vi "CRYAuto Save.vi"(0 "Setup in":T1={"No.VI"=0, "Category"="", "StepName"="", "Seq setup flattened"="", "Comment"="", "Steps config."=[], "Jump config"=[], "Start"=0.0, "Increment"=0.0, "Name"="Pa", "Unit"="Pa", "Y data"=1, "Y prefix"="", "Y dB ref"=1.0, "Y unit"="", "Repeat State Array"=[]} {"Repeat State Array"."Start" format="%#_5g"; "Y dB ref" format="%.1f"; "Y data" items=["dB", "Lin"]; "Start" format="%#_5g"}, 5 "Data in":T6 {"Z data" items=["dB", "Lin"]; "X data" items=["dB", "Lin"]; "Y data" items=["dB", "Lin"]; "Z dB ref" format="%.1f"; "Z axis" items=["Log", "Lin"]; "X dB ref" format="%.1f"; "X axis" items=["Log", "Lin"]; "Y axis" items=["Log", "Lin"]; "Y dB ref" format="%.1f"; "Curve"."z" format="%.2f"; "Curve"."y" format="%.2f"; "Curve"."x" format="%.2f"}, 7 "Results in":T2 {"Margin" format="%.2f"}, 9 "Seq Setup in":string, 11 "Step name":string, 12 "Hardware in":string, 13 "Calibration in":string) -> (3 "Types Out":string[](array[string]), 4 "Inserted Names Out":string[](array[string]), 6 "Data out":T6 {"Z data" items=["dB", "Lin"]; "X data" items=["dB", "Lin"]; "Y data" items=["dB", "Lin"]; "Z dB ref" format="%.1f"; "Z axis" items=["Log", "Lin"]; "X dB ref" format="%.1f"; "X axis" items=["Log", "Lin"]; "Y axis" items=["Log", "Lin"]; "Y dB ref" format="%.1f"; "Curve"."z" format="%.2f"; "Curve"."y" format="%.2f"; "Curve"."x" format="%.2f"}, 8 "Results out":T2 {"Margin" format="%.2f"}, 10 "Wave out":T4 {"Y dB ref" format="%.1f"; "Y axis" items=["Log", "Lin"]; "Y data" items=["dB", "Lin"]; "X data" items=["dB", "Lin"]})   [LabVIEW 2013]
uses:
  Typedef Control/CRYData Cluster Array.ctl
  Typedef Control/CRYData Cluster.ctl
  Typedef Control/CRYResult Cluster Array.ctl
  Typedef Control/CRYResult Cluster.ctl
  Typedef Control/CRYWaveform Cluster Array.ctl
  Typedef Control/CRYWaveform Cluster.ctl
  Typedef Control/CRYStep.ctl
  Data/CRYData & result stacks global.vi
  CRYMainGlobal.vi
  Calibration/SubVI/CRYCal Global.vi
  CRYProject/CRYProject Editor Global.vi
panel:
  out "Channel":i32
  out "filepath":string caption="Saving to file:"
  in  "Display Step":bool=TRUE
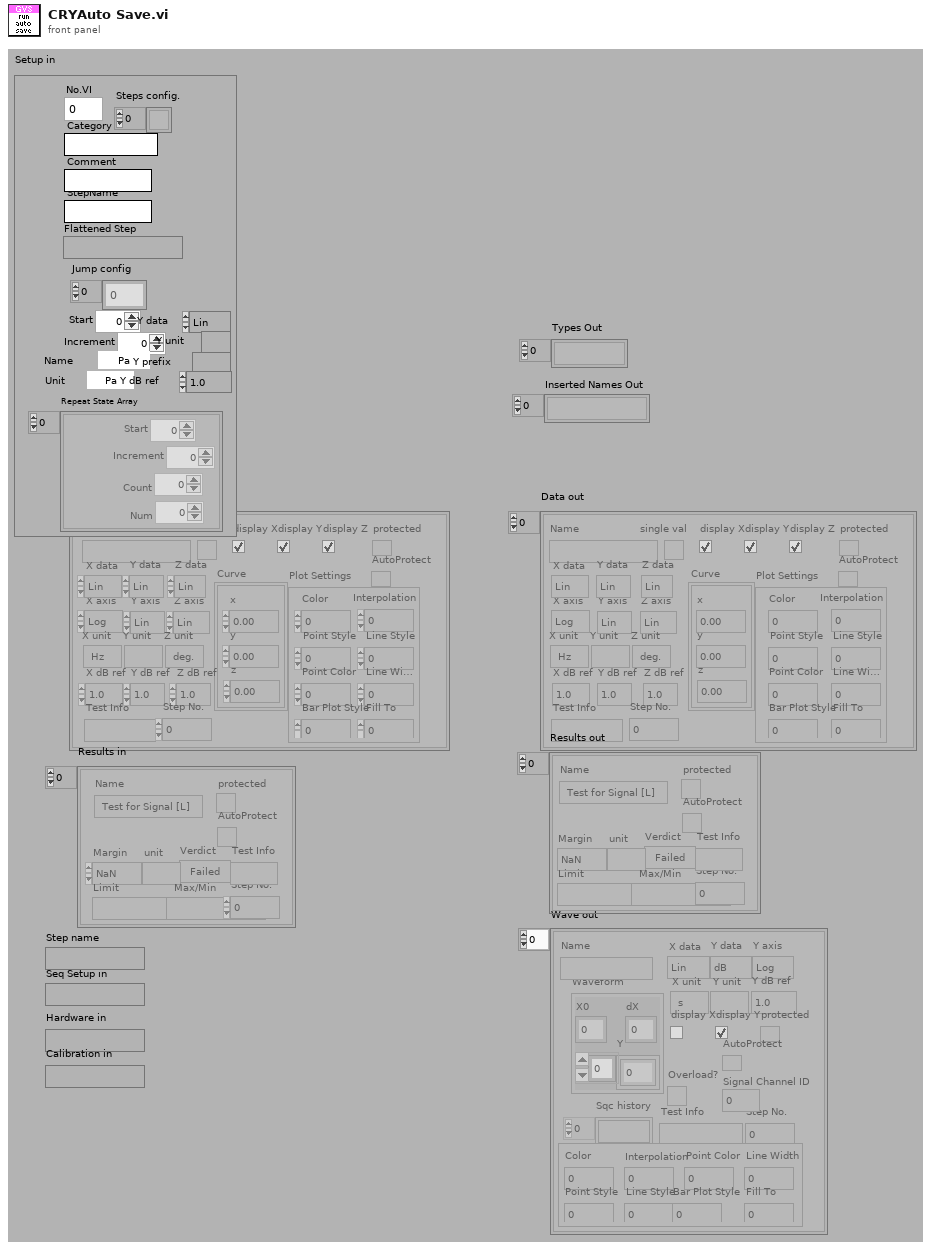
[diagram p1: front panel]
types:
  T1 = typedef "CRYStep.ctl" = cluster{"No.VI":i32, "Category":string, "StepName":string, "Seq setup flattened":string, "Comment":string, "Steps config.":bool[], "Jump config":i32[], "Start":dbl, "Increment":dbl, "Name":string, "Unit":string, "Y data":u16, "Y prefix":string, "Y dB ref":dbl, "Y unit":string, "Repeat State Array":cluster{"Start":dbl, "Increment":dbl, "Count":i32, "Num":i32}[]}
  T2 = typedef "CRYResult Cluster Array.ctl" = T3[]
  T3 = typedef "CRYResult Cluster.ctl" = cluster{"Name":string, "Margin":dbl, "unit":string, "Verdict":bool, "Limit":string, "Max/Min":string, "protected":bool, "Step No.":i32, "Test Info":string, "AutoProtect":bool}
  T4 = typedef "CRYWaveform Cluster Array.ctl" = T5[]
  T5 = typedef "CRYWaveform Cluster.ctl" = cluster{"Waveform":cluster{"X0":dbl, "dX":dbl, "Y":sgl[]}, "X data":u16, "Y data":u16, "Y axis":u16, "X unit":string, "Y unit":string, "Y dB ref":dbl, "display Y":bool, "display X":bool, "Overload?":bool, "Test Info":string, "Step No.":i32, "Name":string, "protected":bool, "Sqc history":string[], "Signal Channel ID":i32, "Plot Settings":cluster{"Color":u32, "Interpolation":u8, "Point Style":u8, "Line Style":u8, "Point Color":u32, "Line Width":u8, "Bar Plot Style":u8, "Fill To":i16}, "AutoProtect":bool}
  T6 = typedef "CRYData Cluster Array.ctl" = T7[]
  T7 = typedef "CRYData Cluster.ctl" = cluster{"Name":string, "Curve":cluster{"x":dbl, "y":dbl, "z":dbl}[], "X data":u16, "Y data":u16, "Z data":u16, "X axis":u16, "Y axis":u16, "Z axis":u16, "X unit":string, "Y unit":string, "Z unit":string, "X dB ref":dbl, "Y dB ref":dbl, "Z dB ref":dbl, "single val":bool, "protected":bool, "display X":bool, "display Y":bool, "display Z":bool, "Test Info":string, "Step No.":i32, "Plot Settings":cluster{"Color":u32, "Interpolation":u8, "Point Style":u8, "Line Style":u8, "Point Color":u32, "Line Width":u8, "Bar Plot Style":u8, "Fill To":i16}, "AutoProtect":bool}
  T8 = enum16{"OK", "Yes", "YesNo", "YesNoCancel", "ReplaceAppend"}
  T9 = typedef "CRYAuto Save Cluster.ctl" = cluster{"Name":string, "save":enum16{"Data", "Results", "Waveforms"}, "Item Names":string[], "Autosave folder":path, "data format":u16, "filename option":enum16{"auto", "prompt"}, "fn construction":i32[], "layout":enum16{"rows", "columns"}, "notation":enum16{"sci", "float"}, "precision":i32, "prompt comment":bool, "header":enum16{"none", "standard", "custom"}, "custom header":string, "serial no.":bool, "User defined":string, "delimiter":enum16{"tab", "comma", "space", "other"}, "other delim":string, "axes":cluster{"x":bool, "y":bool, "z":bool}, "Time Stamp":bool, "Lot No.":bool, "Operator":bool, "Excel Template":string, "New or Append":u16, "Data":u16, "Help":string, "Tab Value":enum32{"Setting", "Help"}, "UDL or DSN":path, "User Default":bool, "Selector":i32, "Axis":u16, "Value Name":string, "format string":cluster{"dB Format String out":string, "Lin Format String out":string}, "DBPath":path}
  T10 = cluster{"dB Format String out":string, "Lin Format String out":string}
  T11 = cluster{"layout":enum16{"rows", "columns"}, "notation":enum16{"sci", "float"}, "precision":i32, "header":enum16{"none", "standard", "custom"}, "custom header":string, "serial no.":bool, "delimiter":enum16{"tab", "comma", "space", "other"}, "other delim":string, "axes":cluster{"x":bool, "y":bool, "z":bool}, "Lot No.":bool, "Operator":bool, "Time Stamp":bool}
  T12 = typedef "CRYTS.ctl" = cluster{"No.TS":u16, "TS File Path":path, "TS Name":string, "EditStepName":string, "Steps":T1[], "New State":bool, "Change State":bool, "Flattened CurveLib Data":string, "Document Data":string, "EditStepNo":u16, "Operator Start File":string, "Sequence Type":string, "Sequence Language":string}
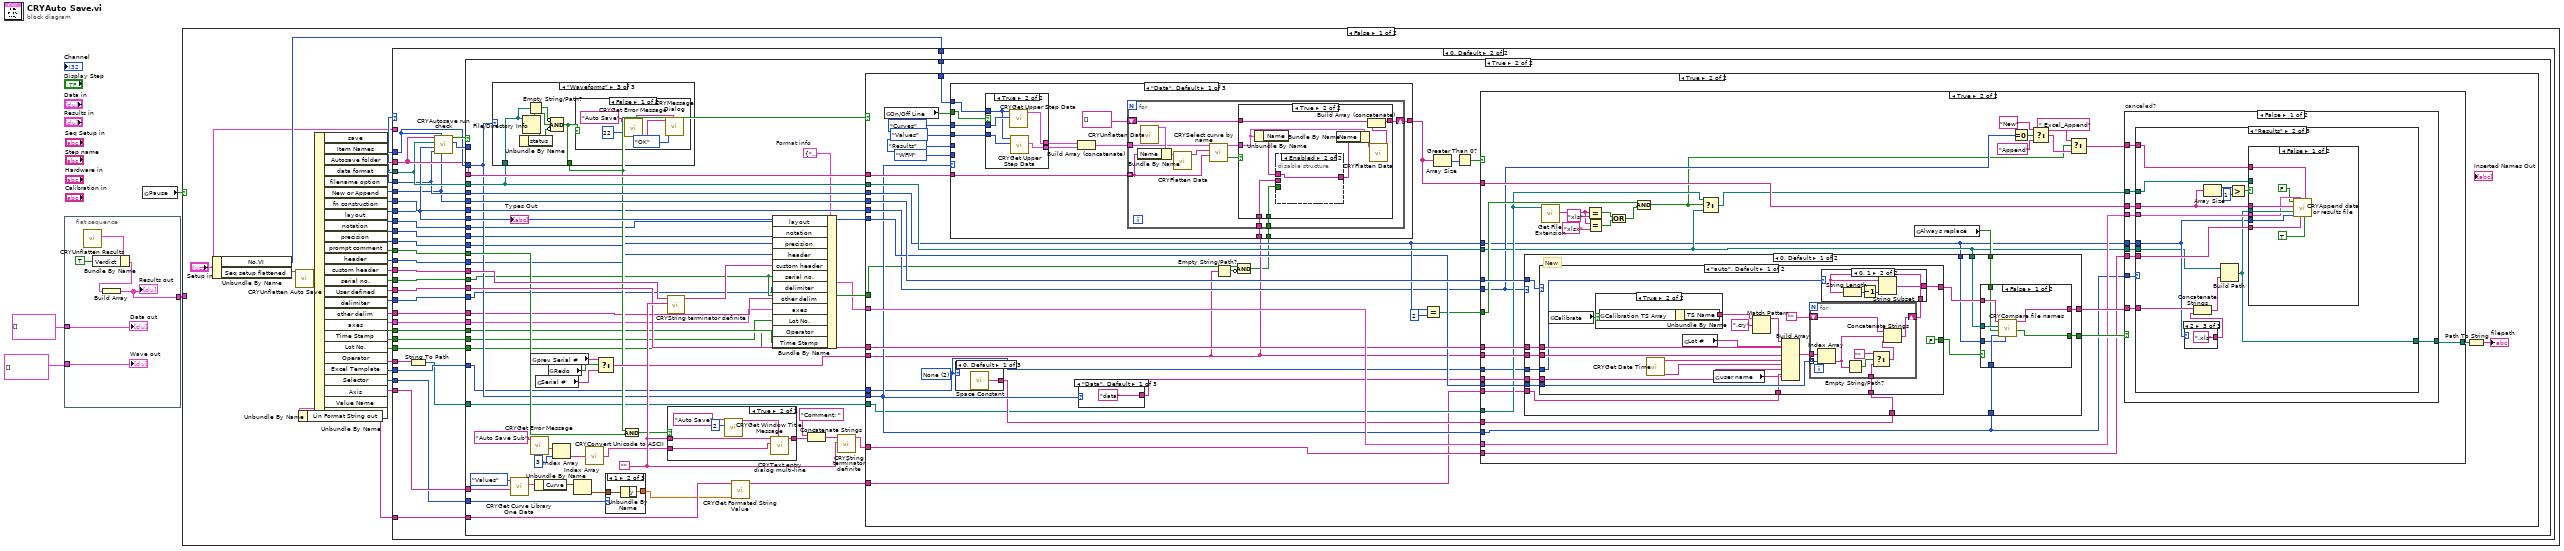
[diagram p0: block diagram]
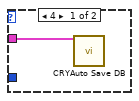
[diagram p2: hidden frame]
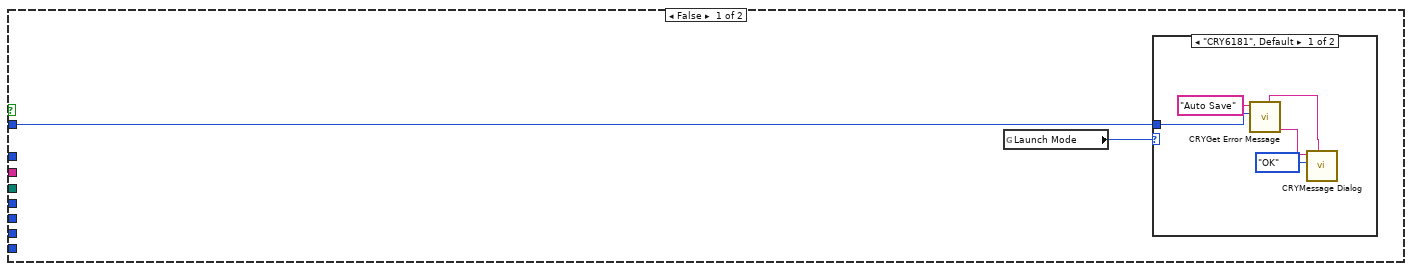
[diagram p3: hidden frame]
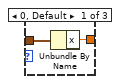
[diagram p5: hidden frame]
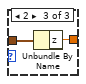
[diagram p6: hidden frame]
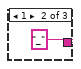
[diagram p8: hidden frame]
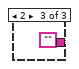
[diagram p9: hidden frame]
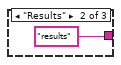
[diagram p10: hidden frame]
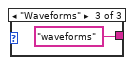
[diagram p11: hidden frame]
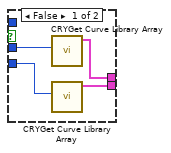
[diagram p12: hidden frame]
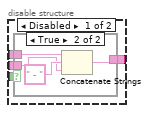
[diagram p14: hidden frame]
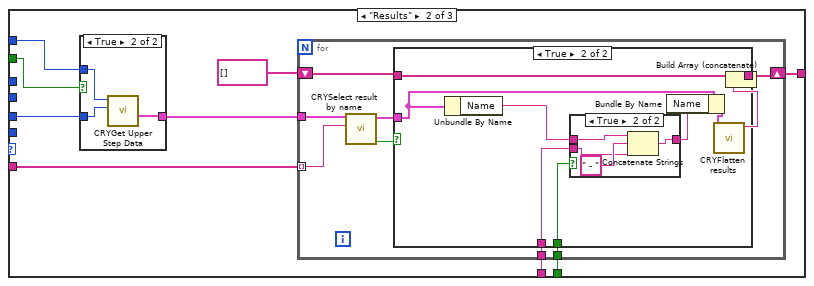
[diagram p16: hidden frame]
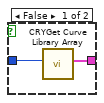
[diagram p17: hidden frame]
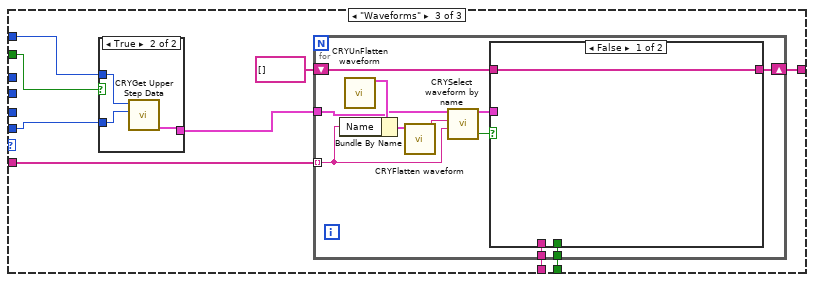
[diagram p20: hidden frame]
diagram:
  n1 = flat-sequence {
    tunnel: T6 [] ("Data out") -> [w7]
    tunnel: [w6] -> w3
    tunnel: T4 [] ("Wave out") -> [w5]
    frame #0 {
      n2 = call "CRYUnflatten Results.vi"() -> ("Result"=w10:T3)  [unwired: 9 in, 2 out]
      n3 = Bundle By Name(cluster=w10, "Verdict"=TRUE) -> (w8:T3)
      n4 = Build Array(w8) -> (w6:T3[])
      "Results out" <- w6
      "Data out" <- w7
      "Wave out" <- w5
    }
  }
  n5 = global read "CRYData & result stacks global.vi" "Pause"() -> (w2:bool)
  n6 = case shown="False" w2 {
    tunnel: w3 -> [_ _]
    frame False {
      n7 = Unbundle By Name("Setup in") -> ("No.VI"=w13:i32, "Seq setup flattened"=w20:string)
      n8 = call "CRYUnflatten Auto Save.vi"("Flatten Auto Save"=w20) -> ("Auto save"=w30:T9)  [unwired: 8 in, 2 out]
      n9 = Unbundle By Name(w30) -> ("save"=w25:enum16{"Data", "Results", "Waveforms"}, "Item Names"=w24:string[], "Autosave folder"=w23:path, "data format"=w12:u16, "filename option"=w21:enum16{"auto", "prompt"}, "New or Append"=w26:u16, "fn construction"=w22:i32[], "layout"=w38:enum16{"rows", "columns"}, "notation"=w39:enum16{"sci", "float"}, "precision"=w40:i32, "prompt comment"=w36:bool, "header"=w41:enum16{"none", "standard", "custom"}, "custom header"=w37:string, "serial no."=w34:bool, "User defined"=w35:string, "delimiter"=w33:enum16{"tab", "comma", "space", "other"}, "other delim"=w32:string, "axes"=w31:cluster{"x":bool, "y":bool, "z":bool}, "Time Stamp"=w29:bool, "Lot No."=w28:bool, "Operator"=w27:bool, "Excel Template"=w18:string, "Selector"=w19:i32, "Axis"=w16:u16, "Value Name"=w17:string, "format string"=w15:T10)
      n10 = Unbundle By Name(w15) -> ("Lin Format String out"=w14:string)
      n11 = case shown="0, Default" w12 {
        tunnel: w41 -> [_ w72]
        tunnel: w40 -> [_ w71]
        tunnel: w39 -> [_ w70]
        tunnel: w38 -> [_ w69]
        tunnel: w37 -> [_ w68]
        tunnel: w36 -> [_ w67]
        tunnel: w35 -> [_ w66]
        tunnel: w34 -> [_ w65]
        tunnel: w33 -> [_ w64]
        tunnel: w32 -> [_ w63]
        tunnel: w31 -> [_ w62]
        tunnel: w29 -> [_ w59]
        tunnel: w28 -> [_ w58]
        tunnel: w27 -> [_ w57]
        tunnel: w26 -> [_ w56]
        tunnel: w25 -> [_ w55]
        tunnel: w24 -> [_ w54]
        tunnel: w23 -> [_ w53]
        tunnel: w22 -> [_ w52]
        tunnel: w12 -> [_ w51]
        tunnel: w21 -> [_ w50]
        tunnel: w19 -> [_ w49]
        tunnel: w18 -> [_ w48]
        tunnel: w17 -> [_ w46]
        tunnel: w16 -> [_ w45]
        tunnel: w14 -> [_ w44]
        tunnel: w13 -> [_ w43]
        tunnel: "Setup in" -> [w42 _]
        frame 4 {
          n12 = call "CRYAuto Save DB.vi"("Setup in"=w42) -> ()  [unwired: 15 in]
        }
        frame 0, Default {
          n13 = String To Path(string=w48) -> (path=w47:path)
          n14 = call "CRYAutosave run check.vi"("filename option"=w50, "save in"=w55, "data format"=w51, "fn construction"=w52, "Autosave folder"=w53, "Item Names"=w54) -> ("number"=w60:i32, "save able?"=w61:bool)  [unwired: 3 in]
          n15 = case shown="True" w61 {
            tunnel: w54 -> [_ w131]
            tunnel: w52 -> [_ w130]
            tunnel: w50 -> [_ w129]
            tunnel: w51 -> [_ w128]
            tunnel: w72 -> [_ w89]
            tunnel: w71 -> [_ w90]
            tunnel: w70 -> [_ w91]
            tunnel: w69 -> [_ w92]
            tunnel: w68 -> [_ w127]
            tunnel: w67 -> [_ w114]
            tunnel: w66 -> [_ w121]
            tunnel: w65 -> [_ w87]
            tunnel: w64 -> [_ w86]
            tunnel: w63 -> [_ w85]
            tunnel: w62 -> [_ w84]
            tunnel: w53 -> [_ w119]
            tunnel: w55 -> [_ w111]
            tunnel: w60 -> [w74 _]
            tunnel: w59 -> [_ w83]
            tunnel: w58 -> [_ w82]
            tunnel: w57 -> [_ w81]
            tunnel: w56 -> [_ w112]
            tunnel: w49 -> [_ w107]
            tunnel: w47 -> [_ w106]
            tunnel: w46 -> [_ w105]
            tunnel: w45 -> [_ w101]
            tunnel: w44 -> [_ w99]
            tunnel: w43 -> [_ w94]
            frame False {
              n16 = global read "CRYMainGlobal.vi" "Launch Mode"() -> (w73:enum32{"CRY6181", "CRY6181 One"})
              n17 = case shown="\"CRY6181\", Default" w73 {
                tunnel: w74 -> [w78 _]
                frame "CRY6181", Default {
                  n18 = call "CRYGet Error Message.vi"("Error No"=w78, "Kind"="Auto Save") -> ("Message Sub 3"=w77:string, "Window Title"=w75:string)  [unwired: 4 in, 4 out]
                  n19 = call "CRYMessage Dialog.vi"("Window Title"=w75, "YesNoCancel"=T8."OK", "Message Content"=w77) -> ()  [unwired: 7 in, 2 out]
                }
                frame "CRY6181 One" {
                }
              }
            }
            frame True {
              w93 = T11 {"layout"=enum."rows", "notation"=enum."sci", "precision"=0, "header"=enum."none", "custom header"="", "serial no."=FALSE, "delimiter"=enum."tab", "other delim"="", "axes"={"x"=FALSE, "y"=FALSE, "z"=FALSE}, "Lot No."=FALSE, "Operator"=FALSE, "Time Stamp"=FALSE}  # Format info
              w123 = ""
              n20 = case shown="\"Waveforms\"" w111 {
                tunnel: w119 -> [w595 w605 w616]
                tunnel: [w594 w606 w617] -> w113
                frame "Data", Default {
                  n21 = File/Directory Info(path=w595) -> (directory=w597:bool, error out=w599:errorcluster)  [unwired: 1 in, 5 out]
                  n22 = Unbundle By Name(w599) -> ("status"=w596:bool)
                  n23 = Empty String/Path?(string/path=w595) -> (empty?=w598:bool)
                  n24 = Compound Arithmetic op=AND(invert w598, w597, invert w596) -> (w594:bool)
                  n25 = case shown="False" w594 {
                    frame False {
                      n26 = call "CRYGet Error Message.vi"("Error No"=20, "Kind"="Auto Save") -> ("Message Sub 3"=w602:string, "Window Title"=w600:string)  [unwired: 4 in, 4 out]
                      n27 = call "CRYMessage Dialog.vi"("Window Title"=w600, "YesNoCancel"=T8."OK", "Message Content"=w602) -> ()  [unwired: 7 in, 2 out]
                    }
                    frame True {
                    }
                  }
                }
                frame "Results" {
                  n28 = File/Directory Info(path=w605) -> (directory=w608:bool, error out=w610:errorcluster)  [unwired: 1 in, 5 out]
                  n29 = Unbundle By Name(w610) -> ("status"=w607:bool)
                  n30 = Empty String/Path?(string/path=w605) -> (empty?=w609:bool)
                  n31 = Compound Arithmetic op=AND(invert w609, w608, invert w607) -> (w606:bool)
                  n32 = case shown="False" w606 {
                    frame False {
                      n33 = call "CRYGet Error Message.vi"("Error No"=21, "Kind"="Auto Save") -> ("Message Sub 3"=w613:string, "Window Title"=w611:string)  [unwired: 4 in, 4 out]
                      n34 = call "CRYMessage Dialog.vi"("Window Title"=w611, "YesNoCancel"=T8."OK", "Message Content"=w613) -> ()  [unwired: 7 in, 2 out]
                    }
                    frame True {
                    }
                  }
                }
                frame "Waveforms" {
                  n35 = File/Directory Info(path=w616) -> (directory=w619:bool, error out=w621:errorcluster)  [unwired: 1 in, 5 out]
                  n36 = Unbundle By Name(w621) -> ("status"=w618:bool)
                  n37 = Empty String/Path?(string/path=w616) -> (empty?=w620:bool)
                  n38 = Compound Arithmetic op=AND(invert w620, w619, invert w618) -> (w617:bool)
                  n39 = case shown="False" w617 {
                    frame False {
                      n40 = call "CRYGet Error Message.vi"("Error No"=22, "Kind"="Auto Save") -> ("Message Sub 3"=w624:string, "Window Title"=w622:string)  [unwired: 4 in, 4 out]
                      n41 = call "CRYMessage Dialog.vi"("Window Title"=w622, "YesNoCancel"=T8."OK", "Message Content"=w624) -> ()  [unwired: 7 in, 2 out]
                    }
                    frame True {
                    }
                  }
                }
              }
              n42 = call "CRYGet Curve Library One Data .vi"("Data Name"=w105, "Type"=enum16{"Curves", "Values", "Results", "WFM"}."Values") -> ("Value"=w103:T7)  [unwired: 3 in, 6 out]
              n43 = call "CRYGet Error Message.vi"("Kind"="Auto Save Sub") -> ("Unicode Message Sub"=w109:string[])  [unwired: 5 in, 5 out]
              n44 = global read "CRYData & result stacks global.vi" "prev Serial #"() -> (w116:string)
              n45 = Unbundle By Name(w103) -> ("Curve"=w102:cluster{"x":dbl, "y":dbl, "z":dbl}[])
              n46 = global read "CRYData & result stacks global.vi" "Serial #"() -> (w117:string)
              n47 = global read "CRYData & result stacks global.vi" "Redo"() -> (w118:bool)
              n48 = Index Array(array=w109, index=3 ("Error No")) -> (element=w96:string)
              n49 = Index Array(array=w102) -> (element=w100:cluster{"x":dbl, "y":dbl, "z":dbl})  [unwired: 1 in]
              n50 = call "CRYConvert Unicode to ASCII.vi"("Unicode"=w96) -> ("ASCII"=w95:string)  [unwired: 4 in]
              n51 = Select(t=w116, s=w118, f=w117) -> (s? t:f=w120:string)
              n52 = case shown="1" w101 {
                tunnel: w100 -> [w133 w135 w137]
                tunnel: [w132 w134 w136] -> w98
                frame 0, Default {
                  n53 = Unbundle By Name(w133) -> ("x"=w132:dbl)
                }
                frame 1 {
                  n54 = Unbundle By Name(w135) -> ("y"=w134:dbl)
                }
                frame 2 {
                  n55 = Unbundle By Name(w137) -> ("z"=w136:dbl)
                }
              }
              n56 = And(x=w113, y=w114) -> (x .and. y?=w115:bool)
              n57 = call "CRYString terminator definite.vi"("Terminator"=w123, "String in"=w127) -> ("String out"=w88:string)  [unwired: 9 in]
              n58 = case shown="True" w115 {
                tunnel: w95 -> [_ w588]
                tunnel: ["" w592] -> w122
                tunnel: w123 -> [_ w593]
                frame False {
                }
                frame True {
                  n59 = call "CRYGet Window Title Message.vi"("No"=2, "Kind"="Auto Save") -> ("Multibyte String"=w589:string)  [unwired: 4 in, 5 out]
                  n60 = call "CRYText entry dialog multi-line.vi"("text"=w593, "Text"=w588, "Title Name"=w589) -> ("text entered"=w592:string)  [unwired: 6 in, 1 out]
                }
              }
              n61 = call "CRYGet Formated String Value.vi"("Value"=w98, "Flattened Format String"=w99) -> ("Unflattened Format string"=w97:string)  [unwired: 9 in]
              n62 = Bundle By Name(cluster=w93, "layout"=w92, "notation"=w91, "precision"=w90, "header"=w89, "custom header"=w88, "serial no."=w87, "delimiter"=w86, "other delim"=w85, "axes"=w84, "Lot No."=w82, "Operator"=w81, "Time Stamp"=w83) -> (w80:T11)
              n63 = Concatenate Strings("Comment: ", w122) -> (w124:string)
              n64 = call "CRYString terminator definite.vi"("Terminator"=w123, "String in"=w124) -> ("String out"=w125:string)  [unwired: 9 in]
              n65 = case shown="True" w113 {
                tunnel: w131 -> [_ w165]
                tunnel: w130 -> [_ w162]
                tunnel: w129 -> [_ w169]
                tunnel: w128 -> [_ w163]
                tunnel: w80 -> [_ w168]
                tunnel: w125 -> [_ w167]
                tunnel: w121 -> [_ w166]
                tunnel: w120 -> [_ w141]
                tunnel: w87 -> [_ w140]
                tunnel: w119 -> [_ w164]
                tunnel: w112 -> [_ w161]
                tunnel: w111 -> [_ w149]
                tunnel: w107 -> [_ w144]
                tunnel: w106 -> [_ w145]
                tunnel: w97 -> [_ w143]
                tunnel: w94 -> [_ w142]
                frame False {
                }
                frame True {
                  (unwired) 2 items=["Space", "Underscores", "None"] ("Selector")
                  n66 = global read "CRYMainGlobal.vi" "On/Off Line"() -> (w147:bool)
                  n67 = case shown="0, Default" w144 {
                    tunnel: [w170 "_" ""] -> w146
                    frame 0, Default {
                      n68 = call <vilib>:"Space Constant.vi"() -> ("String"=w170:string)
                    }
                    frame 1 {
                    }
                    frame 2 {
                    }
                  }
                  n69 = case shown="\"Data\", Default" w149 {
                    tunnel: ["data" "results" "waveforms"] -> w148
                    frame "Data", Default {
                    }
                    frame "Results" {
                    }
                    frame "Waveforms" {
                    }
                  }
                  n70 = Empty String/Path?(string/path=w141) -> (empty?=w139:bool)
                  n71 = Compound Arithmetic op=AND(w140, invert w139) -> (w138:bool)
                  n72 = case shown="\"Data\", Default" w149 {
                    tunnel: w165 -> [w187 w231 w268]
                    tunnel: [w186 w236 w272] -> w160
                    tunnel: w138 -> [w185 w234 w269]
                    tunnel: w141 -> [w184 w235 w270]
                    tunnel: enum16{"Curves", "Values", "Results", "WFM"}."Curves" ("Type") -> [w183 _ _]
                    tunnel: enum16{"Curves", "Values", "Results", "WFM"}."Values" ("Type") -> [w182 _ _]
                    tunnel: enum16{"Curves", "Values", "Results", "WFM"}."Results" ("Type") -> [_ w233 _]
                    tunnel: enum16{"Curves", "Values", "Results", "WFM"}."WFM" ("Type") -> [_ _ w273]
                    tunnel: w142 -> [w177 w229 w266]
                    tunnel: w147 -> [w178 w230 w267]
                    frame "Data", Default {
                      n73 = case shown="True" w178 {
                        tunnel: w183 -> [w191 w196]
                        tunnel: w182 -> [w190 w195]
                        tunnel: [w189 w193] -> w181
                        tunnel: [w188 w192] -> w179
                        tunnel: w177 -> [_ w194]
                        frame False {
                          n74 = call "CRYGet Curve Library Array.vi"("Type In"=w191) -> ("Curve/Value array"=w189:T6)  [unwired: 10 out]
                          n75 = call "CRYGet Curve Library Array.vi"("Type In"=w190) -> ("Curve/Value array"=w188:T6)  [unwired: 10 out]
                        }
                        frame True {
                          n76 = call "CRYGet Upper Step Data.vi"("Type In"=w196, "No.VI"=w194) -> ("Curve array"=w193:T6)  [unwired: 9 out]
                          n77 = call "CRYGet Upper Step Data.vi"("Type In"=w195, "No.VI"=w194) -> ("Value array"=w192:T6)  [unwired: 9 out]
                        }
                      }
                      n78 = Build Array (concatenate)(w181, w179) -> (w180:T6)
                      n79 = for {
                        tunnel: w180 -> [w198]
                        tunnel: w187 -> [w197] mode=indexing
                        shift-right: [w203] -> w186
                        shift-left: string[] [] -> [w204]
                        tunnel: w185 -> [w200]
                        tunnel: w184 -> [w199]
                        n80 = call "CRYUnflatten Data.vi"() -> ("Datum"=w206:T7)  [unwired: 9 in, 2 out]
                        n81 = Bundle By Name(cluster=w206, "Name"=w197) -> (w207:T7)
                        n82 = call "CRYFlatten Data.vi"("Datum"=w207) -> ("Data flattened"=w205:string)  [unwired: 10 in]
                        n83 = call "CRYSelect curve by name.vi"("Curve name desired (just name, if flat data not wired)"=w197, "Curve name desired (flat data)"=w205, "Data array"=w198) -> ("Exists?"=w202:bool, "Desired Curve"=w201:T7)  [unwired: 5 in, 2 out]
                        n84 = case shown="True" w202 {
                          tunnel: w204 -> [w208 w217]
                          tunnel: [w208 w216] -> w203
                          tunnel: w201 -> [_ w211]
                          tunnel: w200 -> [_ w214]
                          tunnel: w199 -> [_ w209]
                          frame False {
                          }
                          frame True {
                            n85 = Unbundle By Name(w211) -> ("Name"=w215:string)
                            n86 = disable-structure shown="Enabled" {
                              disable-tunnel: w215 -> [w221 w227]
                              disable-tunnel: w214 -> [w220 _]
                              disable-tunnel: [w219 w227] -> w210
                              disable-tunnel: w209 -> [w218 _]
                              frame Disabled {
                                n87 = case shown="True" w220 {
                                tunnel: w221 -> [w222 w226]
                                tunnel: w218 -> [_ w223]
                                tunnel: [w222 w225] -> w219
                                frame False {
                                }
                                frame True {
                                n88 = Concatenate Strings(w226, " - " ("Substring"), w223) -> (w225:string)
                                }
                                }
                              }
                              frame Enabled {
                              }
                            }
                            n89 = Bundle By Name(cluster=w211, "Name"=w210) -> (w213:T7)
                            n90 = call "CRYFlatten Data.vi"("Datum"=w213) -> ("Data flattened"=w212:string)  [unwired: 10 in]
                            n91 = Build Array (concatenate)(w217, w212) -> (w216:string[])
                          }
                        }
                      }
                    }
                    frame "Results" {
                      n92 = case shown="True" w230 {
                        tunnel: w233 -> [w238 w241]
                        tunnel: [w237 w239] -> w232
                        tunnel: w229 -> [_ w240]
                        frame False {
                          n93 = call "CRYGet Curve Library Array.vi"("Type In"=w238) -> ("Result array"=w237:T2)  [unwired: 10 out]
                        }
                        frame True {
                          n94 = call "CRYGet Upper Step Data.vi"("Type In"=w241, "No.VI"=w240) -> ("Result array"=w239:T2)  [unwired: 9 out]
                        }
                      }
                      n95 = for {
                        tunnel: w232 -> [w242]
                        tunnel: w231 -> [w249] mode=indexing
                        shift-right: [w247] -> w236
                        shift-left: string[] [] -> [w248]
                        tunnel: w235 -> [w244]
                        tunnel: w234 -> [w243]
                        n96 = call "CRYSelect result by name.vi"("Result name desired"=w249, "Result array"=w242) -> ("Exists?"=w245:bool, "Desired Result"=w246:T3)  [unwired: 8 in]
                        n97 = case shown="True" w245 {
                          tunnel: w248 -> [w250 w259]
                          tunnel: [w250 w258] -> w247
                          tunnel: w246 -> [_ w253]
                          tunnel: w243 -> [_ w256]
                          tunnel: w244 -> [_ w255]
                          frame False {
                          }
                          frame True {
                            n98 = Unbundle By Name(w253) -> ("Name"=w257:string)
                            n99 = case shown="True" w256 {
                              tunnel: w257 -> [w260 w264]
                              tunnel: w255 -> [_ w261]
                              tunnel: [w260 w263] -> w251
                              frame False {
                              }
                              frame True {
                                n100 = Concatenate Strings(w264, " - " ("Substring"), w261) -> (w263:string)
                              }
                            }
                            n101 = Bundle By Name(cluster=w253, "Name"=w251) -> (w252:T3)
                            n102 = call "CRYFlatten results.vi"("Result in"=w252) -> ("Flatten Result"=w254:string)  [unwired: 10 in]
                            n103 = Build Array (concatenate)(w259, w254) -> (w258:string[])
                          }
                        }
                      }
                    }
                    frame "Waveforms" {
                      n104 = case shown="True" w267 {
                        tunnel: w273 -> [w275 w278]
                        tunnel: [w274 w276] -> w271
                        tunnel: w266 -> [_ w277]
                        frame False {
                          n105 = call "CRYGet Curve Library Array.vi"("Type In"=w275) -> ("Waveform Array"=w274:T4)  [unwired: 10 out]
                        }
                        frame True {
                          n106 = call "CRYGet Upper Step Data.vi"("Type In"=w278, "No.VI"=w277) -> ("Waveform Array"=w276:T4)  [unwired: 9 out]
                        }
                      }
                      n107 = for {
                        tunnel: w271 -> [w281]
                        tunnel: w268 -> [w279] mode=indexing
                        shift-right: [w286] -> w272
                        shift-left: string[] [] -> [w287]
                        tunnel: w269 -> [w283]
                        tunnel: w270 -> [w282]
                        n108 = call "CRYUnFlatten waveform.vi"() -> ("Waveform Cluster"=w289:T5)  [unwired: 9 in, 2 out]
                        n109 = Bundle By Name(cluster=w289, "Name"=w279) -> (w280:T5)
                        n110 = call "CRYFlatten waveform.vi"("Waveform Cluster"=w280) -> ("Flatten Waveform"=w288:string)  [unwired: 10 in]
                        n111 = call "CRYSelect waveform by name.vi"("Wave name desired (just name, if flat wave not wired)"=w279, "Wave name desired (flat Wave)"=w288, "Waveform Array"=w281) -> ("Exists?"=w285:bool, "Desired Waveform"=w284:T5)  [unwired: 5 in, 2 out]
                        n112 = case shown="False" w285 {
                          tunnel: w287 -> [w290 w299]
                          tunnel: [w290 w298] -> w286
                          tunnel: w284 -> [_ w293]
                          tunnel: w283 -> [_ w296]
                          tunnel: w282 -> [_ w295]
                          frame False {
                          }
                          frame True {
                            n113 = Unbundle By Name(w293) -> ("Name"=w297:string)
                            n114 = case shown="True" w296 {
                              tunnel: w297 -> [w300 w304]
                              tunnel: w295 -> [_ w301]
                              tunnel: [w300 w303] -> w291
                              frame False {
                              }
                              frame True {
                                n115 = Concatenate Strings(w304, " - " ("Substring"), w301) -> (w303:string)
                              }
                            }
                            n116 = Bundle By Name(cluster=w293, "Name"=w291) -> (w292:T5)
                            n117 = call "CRYFlatten waveform.vi"("Waveform Cluster"=w292) -> ("Flatten Waveform"=w294:string)  [unwired: 10 in]
                            n118 = Build Array (concatenate)(w299, w294) -> (w298:string[])
                          }
                        }
                      }
                    }
                  }
                  n119 = Equal?(x=w163, y=u16 2) -> (x = y?=w150:bool)
                  n120 = Array Size(array=w160) -> (size(s)=w159:i32)
                  n121 = Greater Than 0?(x=w159) -> (x > 0?=w158:bool)
                  n122 = case shown="True" w158 {
                    tunnel: w160 -> [_ w337]
                    tunnel: w164 -> [_ w327]
                    tunnel: w162 -> [_ w349]
                    tunnel: w169 -> [_ w348]
                    tunnel: w163 -> [_ w315]
                    tunnel: w168 -> [_ w345]
                    tunnel: w167 -> [_ w344]
                    tunnel: [path "" w343] -> w157
                    tunnel: w141 -> [_ w342]
                    tunnel: w166 -> [_ w341]
                    tunnel: w161 -> [_ w320]
                    tunnel: w149 -> [w310 w338]
                    tunnel: w150 -> [_ w330]
                    tunnel: w148 -> [_ w339]
                    tunnel: w146 -> [_ w336]
                    tunnel: w145 -> [_ w328]
                    tunnel: w144 -> [_ w317]
                    tunnel: w143 -> [_ w316]
                    frame False {
                      n123 = case shown="\"Waveforms\"" w310 {
                        tunnel: [25 ("Error No") 26 ("Error No") 27 ("Error No")] -> w308
                        frame "Data", Default {
                        }
                        frame "Results" {
                        }
                        frame "Waveforms" {
                        }
                      }
                      n124 = call "CRYGet Error Message.vi"("Error No"=w308, "Kind"="Auto Save") -> ("Message Sub 3"=w307:string, "Window Title"=w305:string)  [unwired: 4 in, 4 out]
                      n125 = call "CRYMessage Dialog.vi"("Window Title"=w305, "YesNoCancel"=T8."OK", "Message Content"=w307) -> ()  [unwired: 7 in, 2 out]
                    }
                    frame True {
                      n126 = call <vilib>:"Get File Extension.vi"("file"=w328) -> ("lowercase file extension"=w334:string)  [unwired: 1 in, 9 out]
                      n127 = Equal?(x=w334, y="xls") -> (x = y?=w332:bool)
                      n128 = Equal?(x=w334, y="xlsx") -> (x = y?=w331:bool)
                      n129 = Or(x=w332, y=w331) -> (x .or. y?=w329:bool)
                      n130 = Compound Arithmetic op=AND(w330, w329) -> (w319:bool)
                      n131 = Select(t=w328, s=w319, f=w327) -> (s? t:f=w326:path)
                      n132 = global read "CRYData & result stacks global.vi" "Always replace"() -> (w340:bool)
                      n133 = case shown="0, Default" w320 {
                        tunnel: w349 -> [w365 w437]
                        tunnel: w348 -> [w364 _]
                        tunnel: [w358 w428] -> w347
                        tunnel: [w357 FALSE ("Cancelled?")] -> w346
                        tunnel: w342 -> [w363 w434]
                        tunnel: w341 -> [w362 w435]
                        tunnel: w339 -> [w361 w436]
                        tunnel: w340 -> [w356 _]
                        tunnel: w327 -> [w355 _]
                        tunnel: w338 -> [w354 _]
                        tunnel: w336 -> [w353 w427]
                        tunnel: w317 -> [w352 w424]
                        tunnel: w316 -> [w351 w423]
                        tunnel: w315 -> [w350 _]
                        frame 0, Default {
                          # "New"
                          n134 = case shown="\"auto\", Default" w364 {
                            tunnel: w365 -> [w392 _]
                            tunnel: [w380 w421] -> w359
                            tunnel: [FALSE ("Cancelled?") w420] -> w360
                            tunnel: w361 -> [w390 _]
                            tunnel: w363 -> [w389 _]
                            tunnel: w362 -> [w388 _]
                            tunnel: w353 -> [w382 _]
                            tunnel: w352 -> [w377 _]
                            tunnel: w351 -> [w376 _]
                            frame "auto", Default {
                              n135 = global read "CRYCal Global.vi" "Calibrate"() -> (w386:bool)
                              n136 = case shown="True" w386 {
                                tunnel: [w400 w401] -> w384
                                frame False {
                                n137 = call "CRYGet Current TS Steps.vi"() -> ("TS Name"=w400:string)  [unwired: 7 in, 4 out]
                                }
                                frame True {
                                n138 = global read "CRYProject Editor Global.vi" "Calibration TS Array"() -> (w402:T12)
                                n139 = Unbundle By Name(w402) -> ("TS Name"=w401:string)
                                }
                              }
                              n140 = call "CRYGet Date Time.vi"() -> ("time"=w378:string, "date"=w379:string)  [unwired: 10 in]
                              n141 = global read "CRYData & result stacks global.vi" "Lot #"() -> (w387:string)
                              n142 = global read "CRYMainGlobal.vi" "user name"() -> (w375:string)
                              n143 = Match Pattern(string=w384, regular expression=".cry") -> (before substring=w383:string)  [unwired: 1 in, 3 out]
                              n144 = Build Array(w383, w387, w388, w389, w379, w378, w390, w376, w375) -> (w393:string[])
                              n145 = for {
                                shift-right: [w408] -> w381
                                shift-left: "" -> [w411]
                                tunnel: w392 -> [w410] mode=indexing
                                tunnel: w393 -> [w409]
                                tunnel: w382 -> [w403]
                                n146 = Index Array(array=w409, index=w410) -> (element=w405:string)
                                n147 = Empty String/Path?(string/path=w405) -> (empty?=w406:bool)
                                n148 = Select(t="", s=w406, f=w403) -> (s? t:f=w404:string)
                                n149 = Concatenate Strings(w411, w405, w404) -> (w408:string)
                              }
                              n150 = case shown="0, 1" w377 {
                                tunnel: w381 -> [w395 w397]
                                tunnel: [w395 w396] -> w380
                                frame Default {
                                }
                                frame 0, 1 {
                                n151 = String Length(string=w397) -> (length=w399:i32)
                                n152 = Decrement(x=w399) -> (x-1=w398:i32)
                                n153 = String Subset(string=w397, length (rest)=w398) -> (substring=w396:string)  [unwired: 1 in]
                                }
                              }
                            }
                            frame "prompt" {
                              n154 = call "CRYGet Error Message.vi"("Kind"="Auto Save Sub") -> ("Unicode Message Sub"=w418:string[])  [unwired: 5 in, 5 out]
                              n155 = Index Array(array=w418, index=4 ("Error No")) -> (element=w413:string)
                              n156 = call "CRYGet Window Title Message.vi"("No"=1, "Kind"="Auto Save") -> ("Multibyte String"=w414:string)  [unwired: 4 in, 5 out]
                              n157 = call "CRYConvert Unicode to ASCII.vi"("Unicode"=w413) -> ("ASCII"=w412:string)  [unwired: 4 in]
                              n158 = call "CRYText entry dialog multi-line.vi"("Text"=w412, "Title Name"=w414) -> ("text entered"=w421:string, "Cancelled?"=w420:bool)  [unwired: 7 in]
                            }
                          }
                          n159 = case shown="False" w360 {
                            selector: w360 -> [_ w374]
                            tunnel: [w370 w374] -> w357
                            tunnel: w359 -> [w372 w373]
                            tunnel: [w369 w373] -> w358
                            tunnel: w356 -> [w368 _]
                            tunnel: w355 -> [w371 _]
                            tunnel: w354 -> [w367 _]
                            tunnel: w350 -> [w366 _]
                            frame False {
                              n160 = call "CRYCompare file names.vi"("data format"=w366, "save"=w367, "Always replace"=w368, "Autosave folder"=w371, "File name"=w372) -> ("Cancelled?"=w370:bool, "File name  out"=w369:string)  [unwired: 3 in, 1 out]
                            }
                            frame True {
                            }
                          }
                        }
                        frame 1 {
                          # "Append"
                          n161 = global read "CRYCal Global.vi" "Calibrate"() -> (w438:bool)
                          n162 = case shown="True" w438 {
                            tunnel: [w447 w448] -> w432
                            frame False {
                              n163 = call "CRYGet Current TS Steps.vi"() -> ("TS Name"=w447:string)  [unwired: 7 in, 4 out]
                            }
                            frame True {
                              n164 = global read "CRYProject Editor Global.vi" "Calibration TS Array"() -> (w449:T12)
                              n165 = Unbundle By Name(w449) -> ("TS Name"=w448:string)
                            }
                          }
                          n166 = call "CRYGet Date Time.vi"() -> ("time"=w425:string, "date"=w426:string)  [unwired: 10 in]
                          n167 = global read "CRYData & result stacks global.vi" "Lot #"() -> (w439:string)
                          n168 = global read "CRYMainGlobal.vi" "user name"() -> (w422:string)
                          n169 = Match Pattern(string=w432, regular expression=".cry") -> (before substring=w430:string)  [unwired: 1 in, 3 out]
                          n170 = Build Array(w430, w439, w435, w434, w426, w425, w436, w423, w422) -> (w440:string[])
                          n171 = for {
                            shift-right: [w455] -> w429
                            shift-left: "" -> [w458]
                            tunnel: w437 -> [w457] mode=indexing
                            tunnel: w440 -> [w456]
                            tunnel: w427 -> [w450]
                            n172 = Index Array(array=w456, index=w457) -> (element=w452:string)
                            n173 = Empty String/Path?(string/path=w452) -> (empty?=w453:bool)
                            n174 = Select(t="", s=w453, f=w450) -> (s? t:f=w451:string)
                            n175 = Concatenate Strings(w458, w452, w451) -> (w455:string)
                          }
                          n176 = case shown="0, 1" w424 {
                            tunnel: w429 -> [w442 w444]
                            tunnel: [w442 w443] -> w428
                            frame Default {
                            }
                            frame 0, 1 {
                              n177 = String Length(string=w444) -> (length=w446:i32)
                              n178 = Decrement(x=w446) -> (x-1=w445:i32)
                              n179 = String Subset(string=w444, length (rest)=w445) -> (substring=w443:string)  [unwired: 1 in]
                            }
                          }
                        }
                      }
                      n180 = Equal To 0?(x=w320) -> (x = 0?=w321:bool)
                      n181 = Select(t="New", s=w321, f="Append") -> (s? t:f=w325:string)
                      n182 = Select(t=" Excel_Append", s=w319, f=w325) -> (s? t:f=w318:string)
                      n183 = case "canceled?" shown="False" w346 {
                        tunnel: w337 -> [w468 _]
                        tunnel: w327 -> [w467 _]
                        tunnel: w347 -> [w466 _]
                        tunnel: w338 -> [w465 _]
                        tunnel: w315 -> [w464 _]
                        tunnel: w345 -> [w463 _]
                        tunnel: w344 -> [w462 _]
                        tunnel: [w461 path ""] -> w343
                        tunnel: w326 -> [w460 _]
                        tunnel: w318 -> [w459 _]
                        frame False {
                          n184 = case shown="\"Results\"" w465 {
                            tunnel: w468 -> [w482 w522 w553]
                            tunnel: w467 -> [w481 w519 w550]
                            tunnel: w466 -> [w480 w530 w560]
                            tunnel: w464 -> [w479 w520 w549]
                            tunnel: w463 -> [w478 w527 w552]
                            tunnel: w462 -> [w477 w526 w551]
                            tunnel: [w476 w525 w554] -> w461
                            tunnel: w460 -> [w470 w517 _]
                            tunnel: w459 -> [w469 w518 _]
                            frame "Data", Default {
                              n185 = case shown="2" w479 {
                                tunnel: [".txt" ".dat" ".xls"] -> w471
                                frame 0, Default {
                                }
                                frame 1 {
                                }
                                frame 2 {
                                }
                              }
                              n186 = Concatenate Strings(w480, w471) -> (w475:string)
                              n187 = Array Size(array=w482) -> (size(s)=w474:i32)
                              n188 = Build Path(base path=w481, name or relative path=w475) -> (appended path=w476:path)
                              n189 = Greater?(x=w474, y=1) -> (0:w472:bool)
                              n190 = case shown="True" w472 {
                                tunnel: w482 -> [w494 w501]
                                tunnel: w476 -> [w493 w500]
                                tunnel: w479 -> [w492 w498]
                                tunnel: w478 -> [w489 w499]
                                tunnel: w477 -> [w491 w497]
                                tunnel: w469 -> [w487 w496]
                                tunnel: w470 -> [w486 w495]
                                frame False {
                                n191 = call "CRYAppend data or results file.vi"("Excel path"=w486, "Is results? (F)"=FALSE, "New/Append"=w487, "Comment"=w491, "Format info"=w489, "data format"=w492, "Datafile path"=w493, "Curves list to save"=w494, "Data/Wave(if true=wave)?"=FALSE) -> ()  [unwired: 2 in, 1 out]
                                }
                                frame True {
                                n192 = case shown="2" w498 {
                                tunnel: w501 -> [w507 w509 w515]
                                tunnel: w500 -> [w506 w508 w512]
                                tunnel: w499 -> [w503 _ w514]
                                tunnel: w497 -> [w504 _ w516]
                                tunnel: w496 -> [_ _ w511]
                                tunnel: w495 -> [_ _ w510]
                                frame 0, Default {
                                n193 = call "CRYExport data to tab-delimited.vi"("Data/Wave(if true=wave)?"=FALSE, "Comment"=w504, "Format info"=w503, "Use format info? (F)"=TRUE, "data series"=w507, "File path (not wired: dialogue)"=w506) -> ()  [unwired: 3 in, 3 out]
                                }
                                frame 1 {
                                n194 = call "CRYMulti curves save.vi"("Array of flattened data clusters"=w509, "Datafile path"=w508) -> ()  [unwired: 10 in]
                                }
                                frame 2 {
                                n195 = call "CRYMulti Excel Export.vi"("Excel path"=w510, "Datafile path"=w512, "New/Append"=w511, "Comment"=w516, "Format info"=w514, "Curves list to save"=w515, "Is results? (T)"=FALSE ("Is results? (F)")) -> ()  [unwired: 4 in, 1 out]
                                }
                                }
                                }
                              }
                            }
                            frame "Results" {
                              n196 = case shown="2" w520 {
                                tunnel: [".txt" ".res" ".xls"] -> w528
                                frame 0, Default {
                                }
                                frame 1 {
                                }
                                frame 2 {
                                }
                              }
                              n197 = Concatenate Strings(w530, w528) -> (w529:string)
                              n198 = Array Size(array=w522) -> (size(s)=w524:i32)
                              n199 = Build Path(base path=w519, name or relative path=w529) -> (appended path=w525:path)
                              n200 = Greater?(x=w524, y=1) -> (0:w521:bool)
                              n201 = case shown="False" w521 {
                                tunnel: w522 -> [w538 w545]
                                tunnel: w520 -> [w534 w541]
                                tunnel: w527 -> [w533 w544]
                                tunnel: w526 -> [w537 w543]
                                tunnel: w525 -> [w536 w542]
                                tunnel: w518 -> [w531 w540]
                                tunnel: w517 -> [_ w539]
                                frame False {
                                n202 = call "CRYAppend data or results file.vi"("Is results? (F)"=TRUE, "New/Append"=w531, "Comment"=w537, "Format info"=w533, "data format"=w534, "Datafile path"=w536, "Curves list to save"=w538, "Data/Wave(if true=wave)?"=FALSE) -> ()  [unwired: 3 in, 1 out]
                                }
                                frame True {
                                n203 = call "CRYResult save as text.vi"("Excel path"=w539, "Comment"=w543, "New/Append"=w540, "File format"=w541, "Format info"=w544, "Path"=w542, "Results stack, flat"=w545) -> ()  [unwired: 5 in]
                                }
                              }
                            }
                            frame "Waveforms" {
                              n204 = case shown="0, Default" w549 {
                                tunnel: [".txt" ".wfm" ".wav"] -> w559
                                frame 0, Default {
                                }
                                frame 1 {
                                }
                                frame 3 {
                                }
                              }
                              n205 = Concatenate Strings(w560, w559) -> (w558:string)
                              n206 = Array Size(array=w553) -> (size(s)=w557:i32)
                              n207 = Build Path(base path=w550, name or relative path=w558) -> (appended path=w554:path)
                              n208 = Greater?(x=w557, y=1) -> (0:w555:bool)
                              n209 = case shown="True" w555 {
                                tunnel: w554 -> [w565 w571]
                                tunnel: w549 -> [w564 w572]
                                tunnel: w553 -> [w566 w570]
                                tunnel: w552 -> [w567 w569]
                                tunnel: w551 -> [w563 w568]
                                frame False {
                                n210 = call "CRYAppend data or results file.vi"("Is results? (F)"=FALSE, "Comment"=w563, "Format info"=w567, "data format"=w564, "Datafile path"=w565, "Curves list to save"=w566, "Data/Wave(if true=wave)?"=TRUE) -> ()  [unwired: 4 in, 1 out]
                                }
                                frame True {
                                n211 = case shown="0, Default" w572 {
                                tunnel: w571 -> [w577 w579 w581]
                                tunnel: w570 -> [w576 w580 w582]
                                tunnel: w569 -> [w575 _ _]
                                tunnel: w568 -> [w574 _ _]
                                frame 0, Default {
                                n212 = call "CRYExport data to tab-delimited.vi"("Data/Wave(if true=wave)?"=TRUE, "Comment"=w574, "Format info"=w575, "Use format info? (F)"=TRUE, "data series"=w576, "File path (not wired: dialogue)"=w577) -> ()  [unwired: 3 in, 3 out]
                                }
                                frame 1 {
                                n213 = call "CRYMulti curves save.vi"("Array of flattened data clusters"=w580, "Datafile path"=w579) -> ()  [unwired: 10 in]
                                }
                                frame 3 {
                                n214 = call "CRYWaveform Autosave.vi"("File path"=w581, "Flatten Wave"=w582) -> ()  [unwired: 10 in]
                                }
                                }
                                }
                              }
                            }
                          }
                        }
                        frame True {
                        }
                      }
                    }
                  }
                  n215 = Path To String(path=w157) -> (string=→"filepath":string)
                }
              }
            }
          }
        }
      }
    }
    frame True {
    }
  }
